vi "Display loading bar.vi"(6 "Previous state":string, 7 "Loading Bar Display":string, 8 "error in (no error)":errorcluster, 9 "Open?":bool, 10 "Previous control access state":string, 11 "ControlsIndicators in":T1) -> (0 "error out":errorcluster, 2 "Previous state":string, 3 "ControlsIndicators out":T1)   [LabVIEW 2019, in "ZenGage v3.0 UI.lvclass"]
uses:
  ZenGage v3.0 UI.lvclass
  Type Definitions/Controls and Indicators/Select a part (combobox).ctl
  Type Definitions/Controls and Indicators/EDL control references.ctl
  Type Definitions/Controls and Indicators/Diagnostics control referencs.ctl
  Type Definitions/Controls and Indicators/Inspection control references.ctl
  Type Definitions/Controls and Indicators/General_Control references.ctl
  Type Definitions/Controls and Indicators/Controls and Indicators Cluster.ctl
  Type Definitions/General/Master sample references.ctl
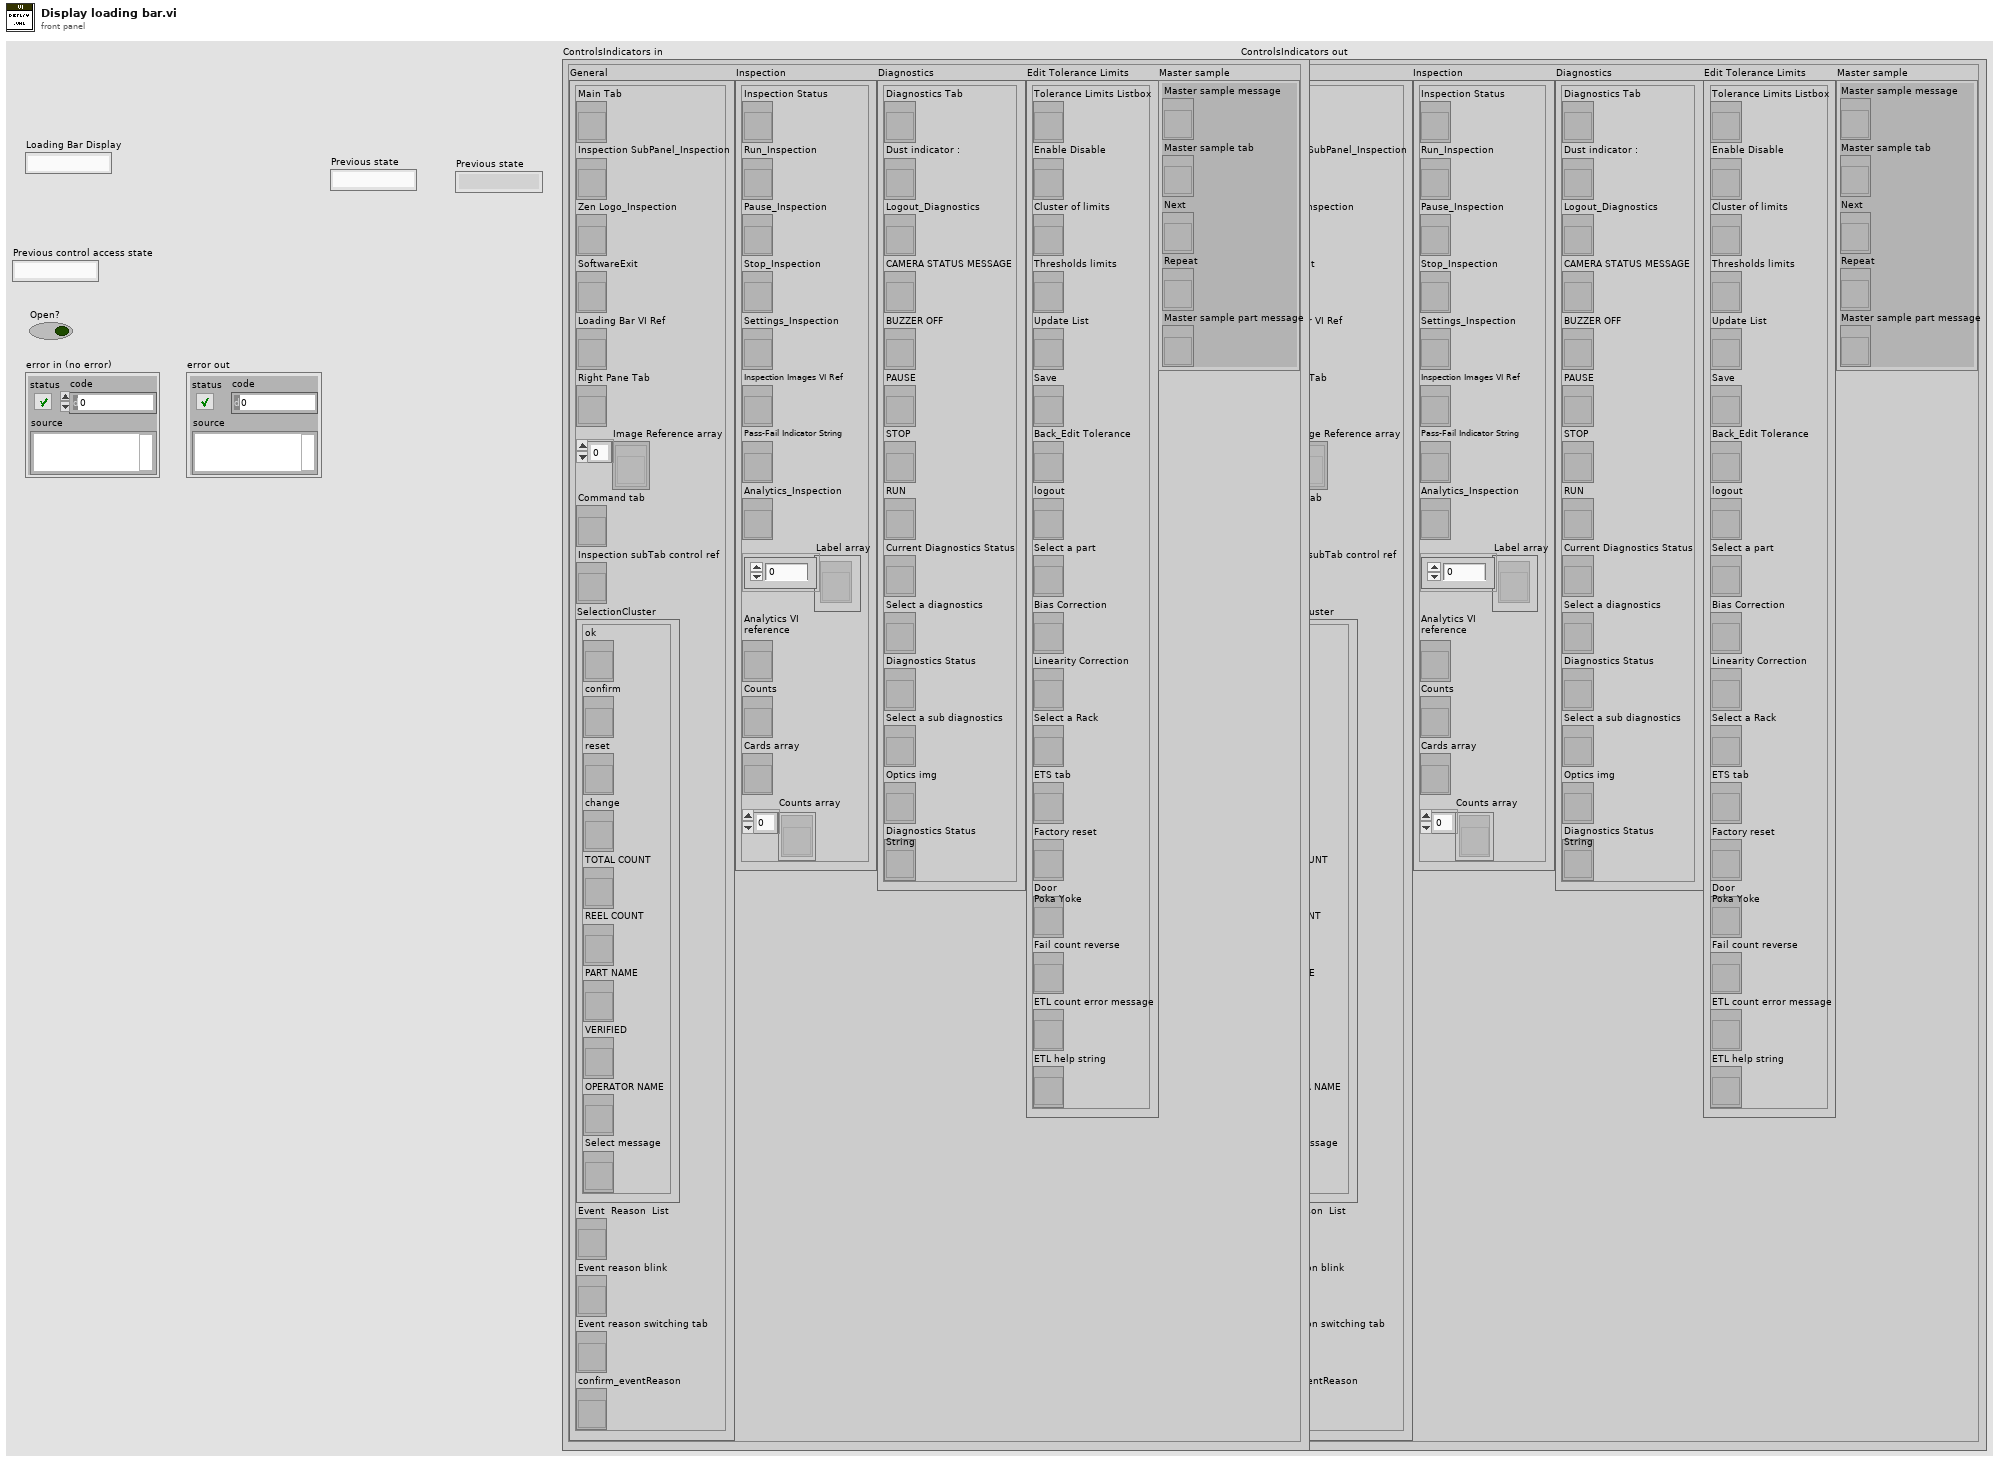
[diagram p1: front panel]
types:
  T1 = typedef "ZenGage v3.0 UI.lvclass/Controls and Indicators Cluster.ctl" = cluster{"General":T2, "Inspection":T3, "Diagnostics":T4, "Edit Tolerance Limits":T5, "Master sample":T6}
  T2 = typedef "ZenGage v3.0 UI.lvclass/General_Control references.ctl" = cluster{"Main Tab":refnum<vi>, "Inspection SubPanel_Inspection":refnum<vi>, "Zen Logo_Inspection":refnum<vi>, "SoftwareExit":refnum<vi>, "Loading Bar VI Ref":refnum<vi>, "Right Pane Tab":refnum<vi>, "Image Reference array":refnum<vi>[], "Command tab":refnum<vi>, "Inspection subTab control ref":refnum<vi>, "SelectionCluster":cluster{"ok":refnum<vi>, "confirm":refnum<vi>, "reset":refnum<vi>, "change":refnum<vi>, "TOTAL COUNT":refnum<vi>, "REEL COUNT":refnum<vi>, "PART NAME":refnum<vi>, "VERIFIED":refnum<vi>, "OPERATOR NAME":refnum<vi>, "Select message":refnum<vi>}, "Event  Reason  List":refnum<vi>, "Event reason blink":refnum<vi>, "Event reason switching tab":refnum<vi>, "confirm_eventReason":refnum<vi>}
  T3 = typedef "ZenGage v3.0 UI.lvclass/Inspection control references.ctl" = cluster{"Inspection Status":refnum<vi>, "Run_Inspection":refnum<vi>, "Pause_Inspection":refnum<vi>, "Stop_Inspection":refnum<vi>, "Settings_Inspection":refnum<vi>, "Inspection Images VI Ref":refnum<vi>, "Pass-Fail Indicator String":refnum<vi>, "Analytics_Inspection":refnum<vi>, "Label array":refnum<vi>[], "Analytics VI\nreference":refnum<vi>, "Counts":refnum<vi>, "Cards array":refnum<vi>, "Counts array":refnum<vi>[]}
  T4 = typedef "ZenGage v3.0 UI.lvclass/Diagnostics control referencs.ctl" = cluster{"Diagnostics Tab":refnum<vi>, "Dust indicator :":refnum<vi>, "Logout_Diagnostics":refnum<vi>, "CAMERA STATUS MESSAGE":refnum<vi>, "BUZZER OFF":refnum<vi>, "PAUSE":refnum<vi>, "STOP":refnum<vi>, "RUN":refnum<vi>, "Current Diagnostics Status":refnum<vi>, "Select a diagnostics":refnum<vi>, "Diagnostics Status":refnum<vi>, "Select a sub diagnostics":refnum<vi>, "Optics img":refnum<vi>, "Diagnostics Status\nString":refnum<vi>}
  T5 = typedef "ZenGage v3.0 UI.lvclass/EDL control references.ctl" = cluster{"Tolerance Limits Listbox":refnum<vi>, "Enable Disable":refnum<vi>, "Cluster of limits":refnum<vi>, "Thresholds limits":refnum<vi>, "Update List":refnum<vi>, "Save":refnum<vi>, "Back_Edit Tolerance":refnum<vi>, "logout":refnum<vi>, "Select a part":refnum<vi>, "Bias Correction":refnum<vi>, "Linearity Correction":refnum<vi>, "Select a Rack":refnum<vi>, "ETS tab":refnum<vi>, "Factory reset":refnum<vi>, "Door\nPoka Yoke":refnum<vi>, "Fail count reverse":refnum<vi>, "ETL count error message":refnum<vi>, "ETL help string":refnum<vi>}
  T6 = typedef "Master sample references.ctl" = cluster{"Master sample message":refnum<vi>, "Master sample tab":refnum<vi>, "Next":refnum<vi>, "Repeat":refnum<vi>, "Master sample part message":refnum<vi>}
  T7 = enum32{"Invalid", "Standard", "Closed", "Hidden", "Minimized", "Maximized"}
  T8 = enum32{"Analytics", "Blank", "Diagnostics", "Run", "Edit Tolerance Settings"}
  T9 = enum8{"Enabled", "Disabled", "Disabled and Grayed Out"}
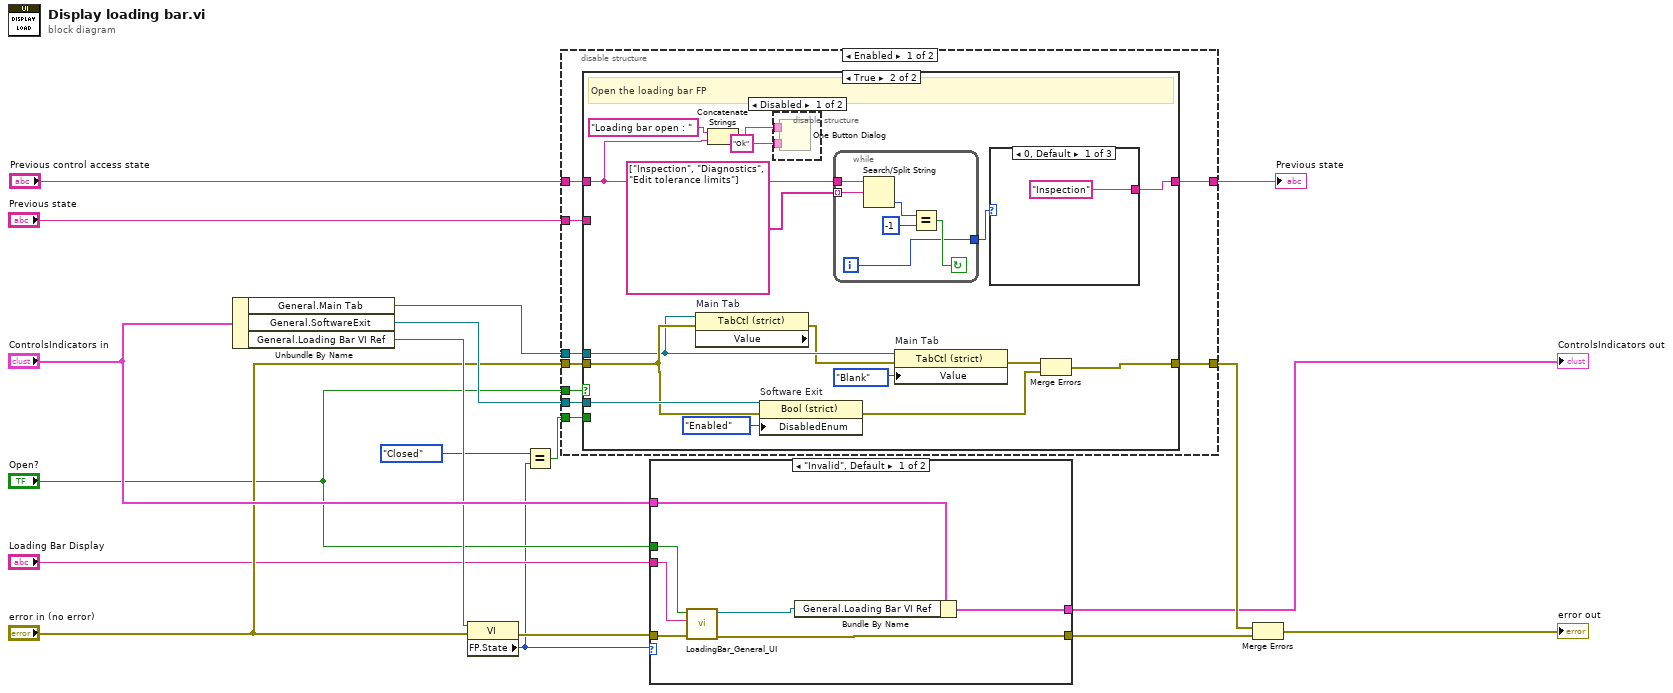
[diagram p0: block diagram]
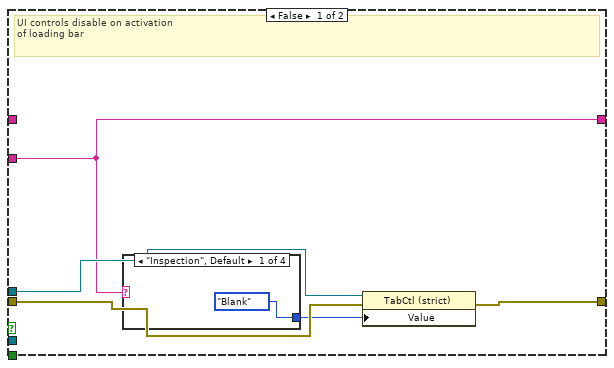
[diagram p2: hidden frame]
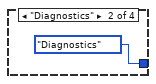
[diagram p3: hidden frame]
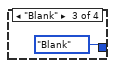
[diagram p4: hidden frame]
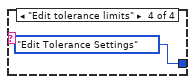
[diagram p5: hidden frame]
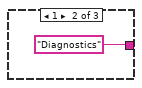
[diagram p7: hidden frame]
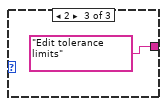
[diagram p8: hidden frame]
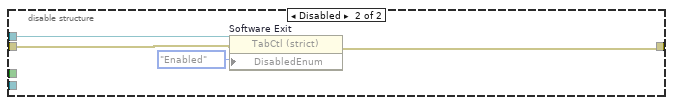
[diagram p9: hidden frame]
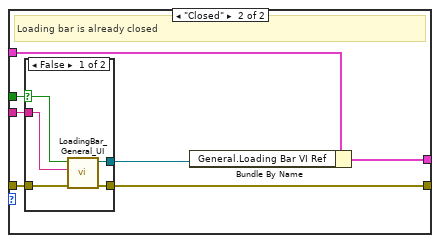
[diagram p10: hidden frame]
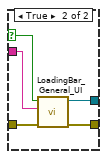
[diagram p11: hidden frame]
diagram:
  n1 = Unbundle By Name("ControlsIndicators in") -> ("General.Main Tab"=w8:refnum<vi>, "General.SoftwareExit"=w13:refnum<vi>, "General.Loading Bar VI Ref"=w14:refnum<vi>)
  n2 = property class="VI"(reference=w14, error in="error in (no error)") -> (error out=w9:errorcluster, "FP.State"=w6:T7)  [unwired: 1 out]
  n3 = Equal?(x=T7."Closed", y=w6) -> (x = y?=w4:bool)
  n4 = disable-structure shown="Enabled" {
    disable-tunnel: [w27 w65] -> w17
    disable-tunnel: w13 -> [w26 _]
    disable-tunnel: "error in (no error)" -> [w25 w66]
    disable-tunnel: "Open?" -> [w24 _]
    disable-tunnel: w8 -> [w23 w64]
    disable-tunnel: "Previous state" -> [w22 _]
    disable-tunnel: w4 -> [w21 _]
    disable-tunnel: "Previous control access state" -> [w20 _]
    disable-tunnel: [w19 _] -> w2
    frame Enabled {
      n5 = case shown="True" w24 {
        tunnel: w25 -> [w31 w44]
        tunnel: [w30 w49] -> w27
        tunnel: w23 -> [w32 w43]
        tunnel: w26 -> [_ w48]
        tunnel: w22 -> [w28 _]
        tunnel: w21 -> [_ _]
        tunnel: w20 -> [_ w38]
        tunnel: [w28 w45] -> w19
        frame False {
          # "UI controls disable on activation\nof loading bar"
          n6 = case shown="\"Inspection\", Default" w28 {
            tunnel: [T8."Blank" ("Value") T8."Diagnostics" ("Value") T8."Blank" ("Value") T8."Edit Tolerance Settings" ("Value")] -> w29
            frame "Inspection", Default {
            }
            frame "Diagnostics" {
            }
            frame "Blank" {
            }
            frame "Edit tolerance limits" {
            }
          }
          n7 = property class="TabCtl (strict)"(reference=w32, error in=w31, "Value"=w29) -> (error out=w30:errorcluster)  [unwired: 1 out]
        }
        frame True {
          # "Open the loading bar FP"
          n8 = property on="Main Tab" class="TabCtl (strict)" props=["Value"](reference=w43, error in=w44) -> (error out=w42:errorcluster)  [unwired: 2 out]
          n9 = Concatenate Strings("Loading bar open : " ("message"), w38) -> (w39:string)
          n10 = property on="Software Exit" class="Bool (strict)"(reference=w48, error in=w44, "DisabledEnum"=T9."Enabled" ("Disabled")) -> (error out=w50:errorcluster)  [unwired: 1 out]
          n11 = disable-structure shown="Disabled" {
            disable-tunnel: w39 -> [w54 _]
            disable-tunnel: "Ok" ("button name (\"OK\")") -> [w53 _]
            frame Disabled {
              n12 = One Button Dialog(message=w54, button name ("OK")=w53) -> ()  [unwired: 1 out]
            }
            frame Enabled {
            }
          }
          n13 = while {
            tunnel: w38 -> [w63]
            tunnel: string[] ["Inspection", "Diagnostics", "Edit tolerance limits"] -> [w62] mode=indexing
            tunnel: [w58] -> w46
            i -> [w58]
            stop <- w59 continue-if-true
            n14 = Search/Split String(string=w63, search string/char (-)=w62) -> (offset of match=w61:i32)  [unwired: 1 in, 2 out]
            n15 = Equal?(x=w61, y=-1) -> (x = y?=w59:bool)
          }
          n16 = property on="Main Tab" class="TabCtl (strict)"(reference=w43, error in=w42, "Value"=T8."Blank") -> (error out=w41:errorcluster)  [unwired: 1 out]
          n17 = case shown="0, Default" w46 {
            tunnel: ["Inspection" "Diagnostics" "Edit tolerance limits"] -> w45
            frame 0, Default {
            }
            frame 1 {
            }
            frame 2 {
            }
          }
          n18 = Merge Errors(w41, w50) -> (w49:errorcluster)
        }
      }
    }
    frame Disabled {
      n19 = property on="Software Exit" class="TabCtl (strict)"(reference=w64, error in=w66, "DisabledEnum"=T9."Enabled" ("Disabled")) -> (error out=w65:errorcluster)  [unwired: 1 out]
    }
  }
  "Previous state" <- w2
  n20 = case shown="\"Invalid\", Default" w6 {
    tunnel: [w74 w81] -> w15
    tunnel: "Loading Bar Display" -> [w73 w79]
    tunnel: "Open?" -> [w70 w80]
    tunnel: "ControlsIndicators in" -> [w72 w78]
    tunnel: [w69 w77] -> w1
    tunnel: w9 -> [w68 w75]
    frame "Invalid", Default {
      n21 = call "LoadingBar_General_UI.vi"("error in (no error)"=w68, "String\n to be displayed"=w73, "Display?"=w70) -> ("error out"=w74:errorcluster, "Loading Bar VI\nRef"=w71:refnum<vi>)  [unwired: 7 in]
      n22 = Bundle By Name(cluster=w72, "General.Loading Bar VI Ref"=w71) -> (w69:T1)
    }
    frame "Closed" {
      # "Loading bar is already closed"
      n23 = case shown="False" w80 {
        selector: w80 -> [w85 w89]
        tunnel: [w86 w91] -> w81
        tunnel: w79 -> [w83 w90]
        tunnel: [w84 w88] -> w76
        tunnel: w75 -> [w82 w87]
        frame False {
          n24 = call "LoadingBar_General_UI.vi"("error in (no error)"=w82, "String\n to be displayed"=w83, "Display?"=w85) -> ("error out"=w86:errorcluster, "Loading Bar VI\nRef"=w84:refnum<vi>)  [unwired: 7 in]
        }
        frame True {
          n25 = call "LoadingBar_General_UI.vi"("error in (no error)"=w87, "String\n to be displayed"=w90, "Display?"=w89) -> ("error out"=w91:errorcluster, "Loading Bar VI\nRef"=w88:refnum<vi>)  [unwired: 7 in]
        }
      }
      n26 = Bundle By Name(cluster=w78, "General.Loading Bar VI Ref"=w76) -> (w77:T1)
    }
  }
  "ControlsIndicators out" <- w1
  n27 = Merge Errors(w17, w15) -> (→"error out":errorcluster)
